vi "Show Measurements.vi"(0 "InfluxDB in":refnum<class "Client.lvclass">, 5 "Database name":string, 11 "error in (no error)":errorcluster) -> (4 "InfluxDB out":refnum<class "Client.lvclass">, 6 "Measurement names":string[](array[string]), 15 "error out":errorcluster)   [LabVIEW 2018, in "InfluxDB Client.lvlib" / "Client.lvclass"]
doc: "Creates a database."
uses:
  Client.lvclass
  Results/Results.lvclass
  Results/Results.lvclass/Results.ctl
  Result/Result.lvclass/Result.ctl
  Series/Series.lvclass/Series.ctl
  <vilib>/LVH/i3 JSON/i3-json.lvlib
  Result/Result.lvclass
  Series/Series.lvclass
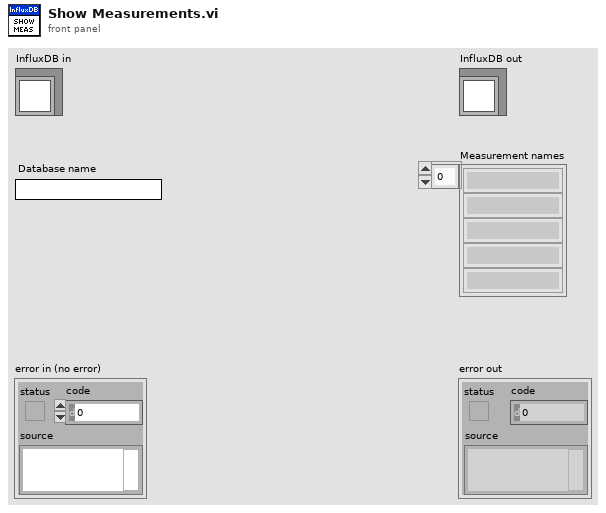
[diagram p1: front panel]
types:
  T1 = typedef "Dictionary Object RefNum__ogtk.ctl" = refnum<k1>
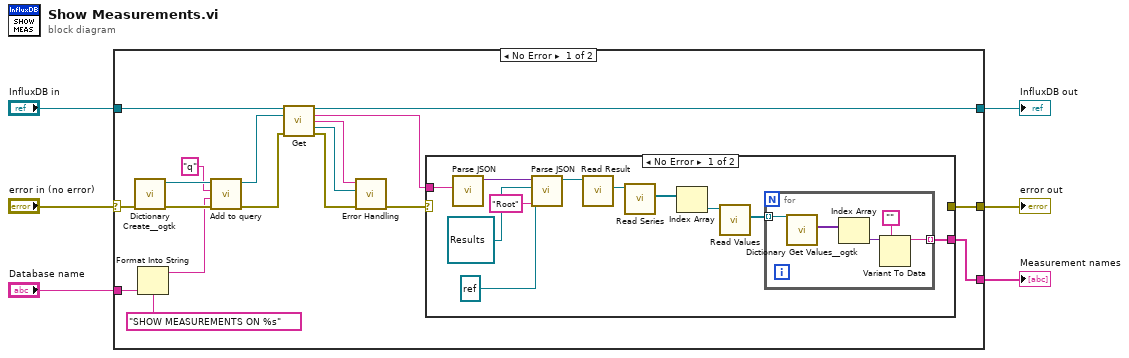
[diagram p0: block diagram]
diagram:
  n1 = case shown="No Error" "error in (no error)" {
    selector: "error in (no error)" -> [w18 w42]
    tunnel: [w23 w43] -> w4
    tunnel: "InfluxDB in" -> [w24 w43]
    tunnel: [w11 w42] -> w2
    tunnel: [w10 _] -> w3
    tunnel: "Database name" -> [w8 _]
    frame No Error {
      n2 = call <userlib>:"Dictionary Create__ogtk.vi"("error in (no error)"=w18) -> ("error out"=w17:errorcluster, "dictionary out"=w22:T1)  [unwired: 9 in]
      n3 = Format Into String(format string="SHOW MEASUREMENTS ON %s" ("Username"), w8) -> (resulting string=w7:string)  [unwired: 2 in, 1 out]
      n4 = call "Add to query.vi"("error in (no error)"=w17, "Value"=w7, "Parameter"="q" ("String"), "Query in"=w22) -> ("error out"=w19:errorcluster, "Query out"=w20:T1)  [unwired: 6 in]
      n5 = call "Get.vi"("InfluxDB Client in"=w24, "Query"=w20, "error in (no error)"=w19) -> ("InfluxDB Client out"=w23:refnum<class "Client.lvclass">, "body"=w16:string, "Status code"=w15:string, "Headers"=w13:T1, "error out"=w14:errorcluster)  [unwired: 8 in]
      n6 = call "Error Handling.vi"("error in (no error)"=w14, "HTTP headers"=w13, "HTTP status code"=w15) -> ("error out"=w12:errorcluster)  [unwired: 8 in]
      n7 = case shown="No Error" w12 {
        selector: w12 -> [_ w41]
        tunnel: w16 -> [w35 _]
        tunnel: [_ w41] -> w11
        tunnel: [w25 _] -> w10
        frame No Error {
          n8 = call <vilib>:"Parse JSON.vi"("JSON String"=w35) -> ("JSON Tree"=w34:variant)  [unwired: 7 in, 3 out]
          n9 = call <vilib>:"Parse JSON.vi"("Path"="Root", "Log File Ref"=refnum<file> refnum, "Results In"=refnum<class "Results.lvclass"> refnum, "JSON Tree"=w34) -> ("Results Out"=w26:refnum<class "Results.lvclass">)  [unwired: 7 in]
          n10 = call "Read Result.vi"("Results in"=w26) -> ("Result.lvclass"=w27:refnum<class "Result.lvclass">)  [unwired: 9 in, 1 out]
          n11 = call "Read Series.vi"("Result in"=w27) -> ("Series"=w28:refnum<class "Series.lvclass">[])  [unwired: 9 in, 1 out]
          n12 = Index Array(array=w28) -> (element=w29:refnum<class "Series.lvclass">)  [unwired: 1 in]
          n13 = call "Read Values.vi"("Series in"=w29) -> ("Values"=w30:T1[])  [unwired: 9 in, 1 out]
          n14 = for {
            tunnel: w30 -> [w40] mode=indexing
            tunnel: [w36] -> w25 mode=indexing
            n15 = call <userlib>:"Dictionary Get Values__ogtk.vi"("dictionary"=w40) -> ("values"=w39:variant[])  [unwired: 8 in, 2 out]
            n16 = Index Array(array=w39) -> (element=w38:variant)  [unwired: 1 in]
            n17 = Variant To Data(type="", Variant=w38) -> (data=w36:string)  [unwired: 1 in, 1 out]
          }
        }
        frame Error {
        }
      }
    }
    frame Error {
    }
  }
  "error out" <- w2
  "InfluxDB out" <- w4
  "Measurement names" <- w3
